vi "CriticalMain.vi"(8 "error in (no error)":errorcluster) -> (0 "error out":errorcluster)   [LabVIEW 2014]
uses:
  Type Defs/CriticalToFValues.ctl
  Type Defs/PositionSensorData.ctl
  Type Defs/PodState.ctl
  <vilib>/Platform/TimedLoop/XDataNode/timing_clust.ctl
  <vilib>/Platform/TimedLoop/XDataNode/nitl_modes.ctl
  <vilib>/Platform/TimedLoop/XDataNode/wakeup.ctl
  <vilib>/myRIO/Instrument Drivers/Onboard Devices/Accelerometer/typedefs/Accelerometer Reference.ctl
  <vilib>/myRIO/Common/Instrument Driver Framework/Utilities/typedefs/myRIO Generic Hardware Reference.ctl
  <vilib>/myRIO/Common/Instrument Driver Framework/Utilities/typedefs/Hardware Version Enum.ctl
  <vilib>/myRIO/Common/Instrument Driver Framework/Utilities/typedefs/myRIO v1.0 Reference.ctl
  <vilib>/myRIO/Common/Instrument Driver Framework/Utilities/typedefs/Generic FPGA Reference.ctl
  <vilib>/myRIO/Common/Instrument Driver Framework/myRIO v1.0/Accelerometer/typedefs/Accelerometer Channels List.ctl
  <vilib>/myRIO/Common/Instrument Driver Framework/myRIO v1.0/Accelerometer/typedefs/Accelerometer Channels Enum.ctl
  <vilib>/userdefined/High Color/nirio_resource_hc.ctl
  <vilib>/myRIO/Instrument Drivers/Onboard IO/DIO/typedefs/DIO Reference.ctl
  <vilib>/myRIO/Common/Instrument Driver Framework/myRIO v1.0/DIO/typedefs/DIO Channels List.ctl
  <vilib>/myRIO/Common/Instrument Driver Framework/myRIO v1.0/DIO/typedefs/DIO Channels Enum.ctl
  <vilib>/myRIO/Common/Instrument Driver Framework/Utilities/vis/Is FPGA Ref Available.vi
  <vilib>/myRIO/Common/Instrument Driver Framework/myRIO v1.0/Accelerometer/vis/myRIO v1.1 Open Accelerometer.vi
  <vilib>/myRIO/Instrument Drivers/Onboard Devices/Accelerometer/vis/Read.vi
  <vilib>/myRIO/Common/Instrument Driver Framework/myRIO v1.0/DIO/vis/myRIO v1.1 Open DIO.vi
  <vilib>/myRIO/Instrument Drivers/Onboard IO/DIO/vis/Read.vi
  <vilib>/MakerHub/LINX/Public/Peripherals/Digital/Digital Write N Chans.vi
  <vilib>/myRIO/Common/Instrument Driver Framework/Utilities/vis/Validate Channels.vi
  <vilib>/myRIO/Common/Instrument Driver Framework/myRIO v1.0/Accelerometer/vis/myRIO v1.0 Reserve Accelerometer.vi
  <vilib>/myRIO/Common/Instrument Driver Framework/myRIO v1.0/DIO/vis/myRIO v1.0 Reserve DIO.vi
  <vilib>/MakerHub/LINX/Private/Local IO/LinxDigitalWrite.vi
  <vilib>/MakerHub/LINX/Public/Utilities/Check Channel.vi
  <vilib>/myRIO/Common/Instrument Driver Framework/myRIO v1.0/Resource Manager/vis/myRIO v1.0 Reserve Channel List.vi
  <vilib>/myRIO/Common/Instrument Driver Framework/myRIO v1.0/Accelerometer/vis/myRIO v1.0 Build MUX Configuration Accelerometer.vi
  <vilib>/myRIO/Common/Instrument Driver Framework/myRIO v1.0/DIO/vis/myRIO v1.0 Build MUX Configuration DIO.vi
  <vilib>/MakerHub/LINX/Private/myRIO/Utilities/Get DIO Channel Name.vi
  <vilib>/myRIO/Common/Instrument Driver Framework/myRIO v1.0/Resource Manager/vis/myRIO v1.0 Reserve Channel.vi
  <vilib>/myRIO/Common/Instrument Driver Framework/myRIO v1.0/Resource Manager/vis/myRIO v1.0 Unreserve Channel.vi
  <vilib>/myRIO/Common/Instrument Driver Framework/myRIO v1.0/Resource Manager/vis/myRIO v1.0 Create Configuration List.vi
  <vilib>/myRIO/Common/Instrument Driver Framework/myRIO v1.0/Resource Manager/vis/myRIO v1.0 Build Mutex Name.vi
  <vilib>/MakerHub/LINX/Public/Utilities/Open Local.vi
  <vilib>/Platform/TimedLoop/scheduler/LVUserAPI/_suppVIs/Create_1kHz_TSource.vi
  <vilib>/MakerHub/LINX/Private/Utilties/Generate Error.vi
  <vilib>/Utility/VariantDataType/GetNumericInfo.vi
  <vilib>/Utility/error.llb/Error Cluster From Error Code.vi
  <vilib>/myRIO/Common/Instrument Driver Framework/myRIO v1.0/myRIO v1.1 Open.vi
  <vilib>/myRIO/Common/Instrument Driver Framework/myRIO v1.0/Accelerometer/vis/myRIO v1.0 Get Scaling Constant Accelerometer.vi
  <vilib>/myRIO/Common/Instrument Driver Framework/Utilities/vis/IO Manager.vi
  <vilib>/myRIO/Common/Instrument Driver Framework/Utilities/vis/Configuration Manager.vi
  <vilib>/myRIO/Common/Instrument Driver Framework/myRIO v1.0/myRIO v1.0 Close.vi
  <vilib>/myRIO/Common/Instrument Driver Framework/myRIO v1.0/Accelerometer/vis/myRIO v1.0 Read Accelerometer.vi
  <vilib>/myRIO/Common/Instrument Driver Framework/myRIO v1.0/Resource Manager/vis/myRIO v1.0 Configure IO.vi
  <vilib>/myRIO/Common/Instrument Driver Framework/myRIO v1.0/DIO/vis/myRIO v1.0 Read DIO.vi
  <vilib>/platform/TimedLoop/XDataNode/XDataNode.xnode
  <vilib>/myRIO/Express VI/Onboard Devices/Accelerometer/Accelerometer Express VI.xnode
  <vilib>/myRIO/Instrument Drivers/Onboard Devices/Accelerometer/vis/myRIO Accelerometer Open.xnode
  <vilib>/myRIO/Express VI/Onboard IO/DI/DI Express VI.xnode
  <vilib>/myRIO/Instrument Drivers/Onboard IO/DIO/vis/myRIO DIO Open.xnode
  <vilib>/Platform/TimedLoop/XDataNode/XDNodeRunTimeDep.lvlib
  <vilib>/myRIO/Instrument Drivers/Onboard IO/DIO/DIO.lvlib
  <vilib>/MakerHub/LINX/LMH-LINX.lvlib
  <vilib>/myRIO/Instrument Drivers/Onboard Devices/Accelerometer/Accelerometer.lvlib
panel:
  in  "Release Friction Brakes":bool
  in  "Release Magnetic Brakes":bool
  in  "Force Brakes Close":bool
  in  "Open Brakes":bool
  in  "Levitate":bool
  out "Position Data Lost":u32
  out "ToF Data Lost":u32
  out "Position Sensor Data":T1
  out "Accelerometer Error":bool
  out "Critical ToF Values":T2
  in  "Speed Read":bool
  out "Attempts":i32
  out "Sensor Error Code":u8
  in  "Attempts before Timeout":u16=10
  out "Laser Error":bool
  in  "Reset":bool
  in  "Stop":bool
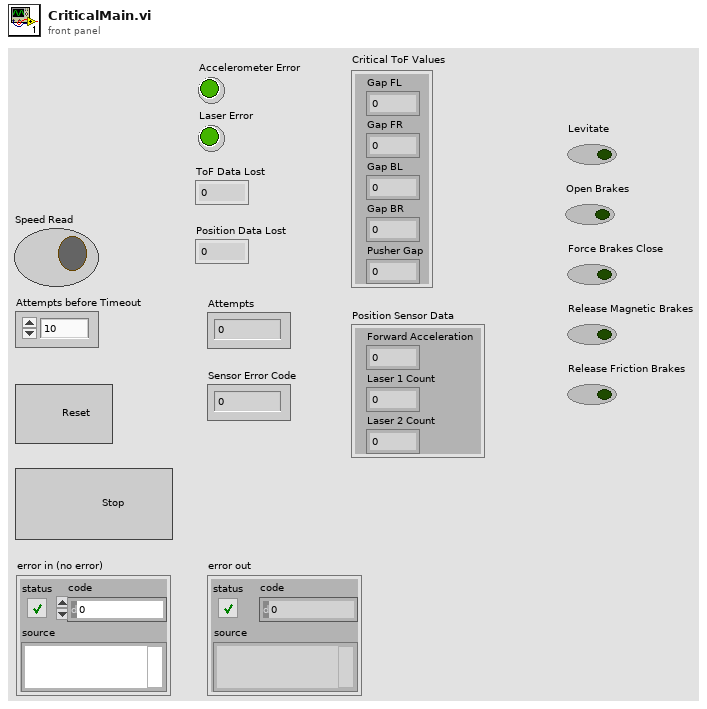
[diagram p1: front panel]
types:
  T1 = typedef "PositionSensorData.ctl" = cluster{"Forward Acceleration":i16, "Laser 1 Count":u16, "Laser 2 Count":u16}
  T2 = typedef "CriticalToFValues.ctl" = cluster{"Gap FL":u8, "Gap FR":u8, "Gap BL":u8, "Gap BR":u8, "Pusher Gap":u8}
  T3 = cluster{"read mode":enum16{"polling", "blocking"}, "write mode":enum16{"polling", "blocking"}}
  T4 = typedef "PodState.ctl" = enum8{"PreFlight", "Accelerating", "Coast", "Brake", "PostFlight"}
  T5 = typedef "LMH-LINX.lvlib/LINX Ref.ctl" = cluster{"IO":T6, "Interface":T7, "LINX Device Config":T8}
  T6 = typedef "LMH-LINX.lvlib/Platform.ctl" = enum16{"Remote", "Local"}
  T7 = typedef "LMH-LINX.lvlib/Interface.ctl" = enum16{"Serial", "TCP"}
  T8 = typedef "LMH-LINX.lvlib/Device.lvlib/LINX Device Config.ctl" = cluster{"Interface":T7, "COM Port":refnum<visa-resource-name>, "TCP Configuration":T9, "Device Family":u8, "Device ID":u8, "Device Name":string, "TCP Ref":refnum<k5>, "Channels":T10}
  T9 = typedef "LMH-LINX.lvlib/Device.lvlib/TCP Config.ctl" = cluster{"IP Address":string, "Port":u16}
  T10 = typedef "LMH-LINX.lvlib/Channels.ctl" = cluster{"DI":u8[], "DO":u8[], "AI":u8[], "AO":u8[], "PWM":u8[], "QE":u8[], "UART":u8[], "I2C 2":u8[], "SPI":u8[], "CAN":u8[], "Servo":u8[], "AI Ref (V)":dbl, "AI Resolution (Bits)":u8, "AO Ref (V)":dbl, "AO Resolution (Bits)":u8}
  T11 = typedef "VL6180 Resource.ctl" = cluster{"I2C Channel":u8, "I2C Slave Address":u8, "Online":bool}
  T12 = typedef "XDNodeRunTimeDep.lvlib/timing_clust.ctl" = cluster{"Expected End [f-1]":u64, "Actual End [f-1]":u64, "Finished Late? [f-1]":bool, "Expected End [i-1]":u64, "Actual End [i-1]":u64, "Finished Late? [i-1]":bool, "Expected Start [i]":u64, "Actual Start [i]":u64, "Expected Start [f]":u64, "Actual Start [f]":u64, "Source Name":string, "Structure Name":string, "Period":i64, "Deadline":i64, "Offset":i64, "Start":i64, "Priority":i32, "Timeout":i32, "Mode":T13, "Wakeup Reason":T14, "Error":errorcluster, "Source Type":string, "Secondary Source Type":string, "Global End Time":u64, "Global Start Time":u64, "Frame Duration":u64, "Iteration Duration":u64, "Assigned CPU":i32, "I/O Scan Engine Mode":u32}
  T13 = typedef "XDNodeRunTimeDep.lvlib/nitl_modes.ctl" = enum32{"No Change", "Process missed periods, maintain original phase", "Discard missed periods, maintain original phase", "Process missed periods, ignore original phase", "Discard missed periods, ignore original phase"}
  T14 = typedef "XDNodeRunTimeDep.lvlib/wakeup.ctl" = enum32{"Normal", "Aborted", "Asynchronous wakeup", "Timing source error", "Timed loop error", "Timeout"}
  T15 = typedef "Accelerometer.lvlib/Accelerometer Reference.ctl" = cluster{"myRIO Reference":T16, "Accelerometer Channels List":T20, "LSB Weight":dbl}
  T16 = typedef "myRIO Generic Hardware Reference.ctl" = cluster{"myRIO Model":T17, "myRIO Hardware Reference":T18}
  T17 = typedef "Hardware Version Enum.ctl" = enum16{"Unknown", "myRIO-1900", "myRIO-1950"}
  T18 = typedef "myRIO v1.0 Reference.ctl" = cluster{"Generic FPGA Reference":T19, "Allow multiple opens":bool}
  T19 = typedef "Generic FPGA Reference.ctl" = refnum<k20>
  T20 = typedef "Accelerometer Channels List.ctl" = T21[]
  T21 = typedef "Accelerometer Channels Enum.ctl" = enum16{"Not Connected", "X-Axis", "Y-Axis", "Z-Axis"}
  T22 = typedef "nirio_resource_hc.ctl" = tag
  T23 = typedef "DIO.lvlib/DIO Reference.ctl" = cluster{"myRIO Reference":T16, "DIO Channels List":T24}
  T24 = typedef "DIO Channels List.ctl" = T25[]
  T25 = typedef "DIO Channels Enum.ctl" = enum16{"Not Connected", "C/DIO0", "C/DIO1", "C/DIO2", "C/DIO3", "C/DIO4", "C/DIO5", "C/DIO6", "C/DIO7", "A/DIO0", "A/DIO1", "A/DIO2", "A/DIO3", "A/DIO4", "A/DIO5", "A/DIO6", "A/DIO7", "A/DIO8", "A/DIO9", "A/DIO10", "A/DIO11", "A/DIO12", "A/DIO13", "A/DIO14", "A/DIO15", "B/DIO0", "B/DIO1", "B/DIO2", "B/DIO3", "B/DIO4", "B/DIO5", "B/DIO6", "B/DIO7", "B/DIO8", "B/DIO9", "B/DIO10", "B/DIO11", "B/DIO12", "B/DIO13", "B/DIO14", "B/DIO15", "LED0", "LED1", "LED2", "LED3", "Button0"}
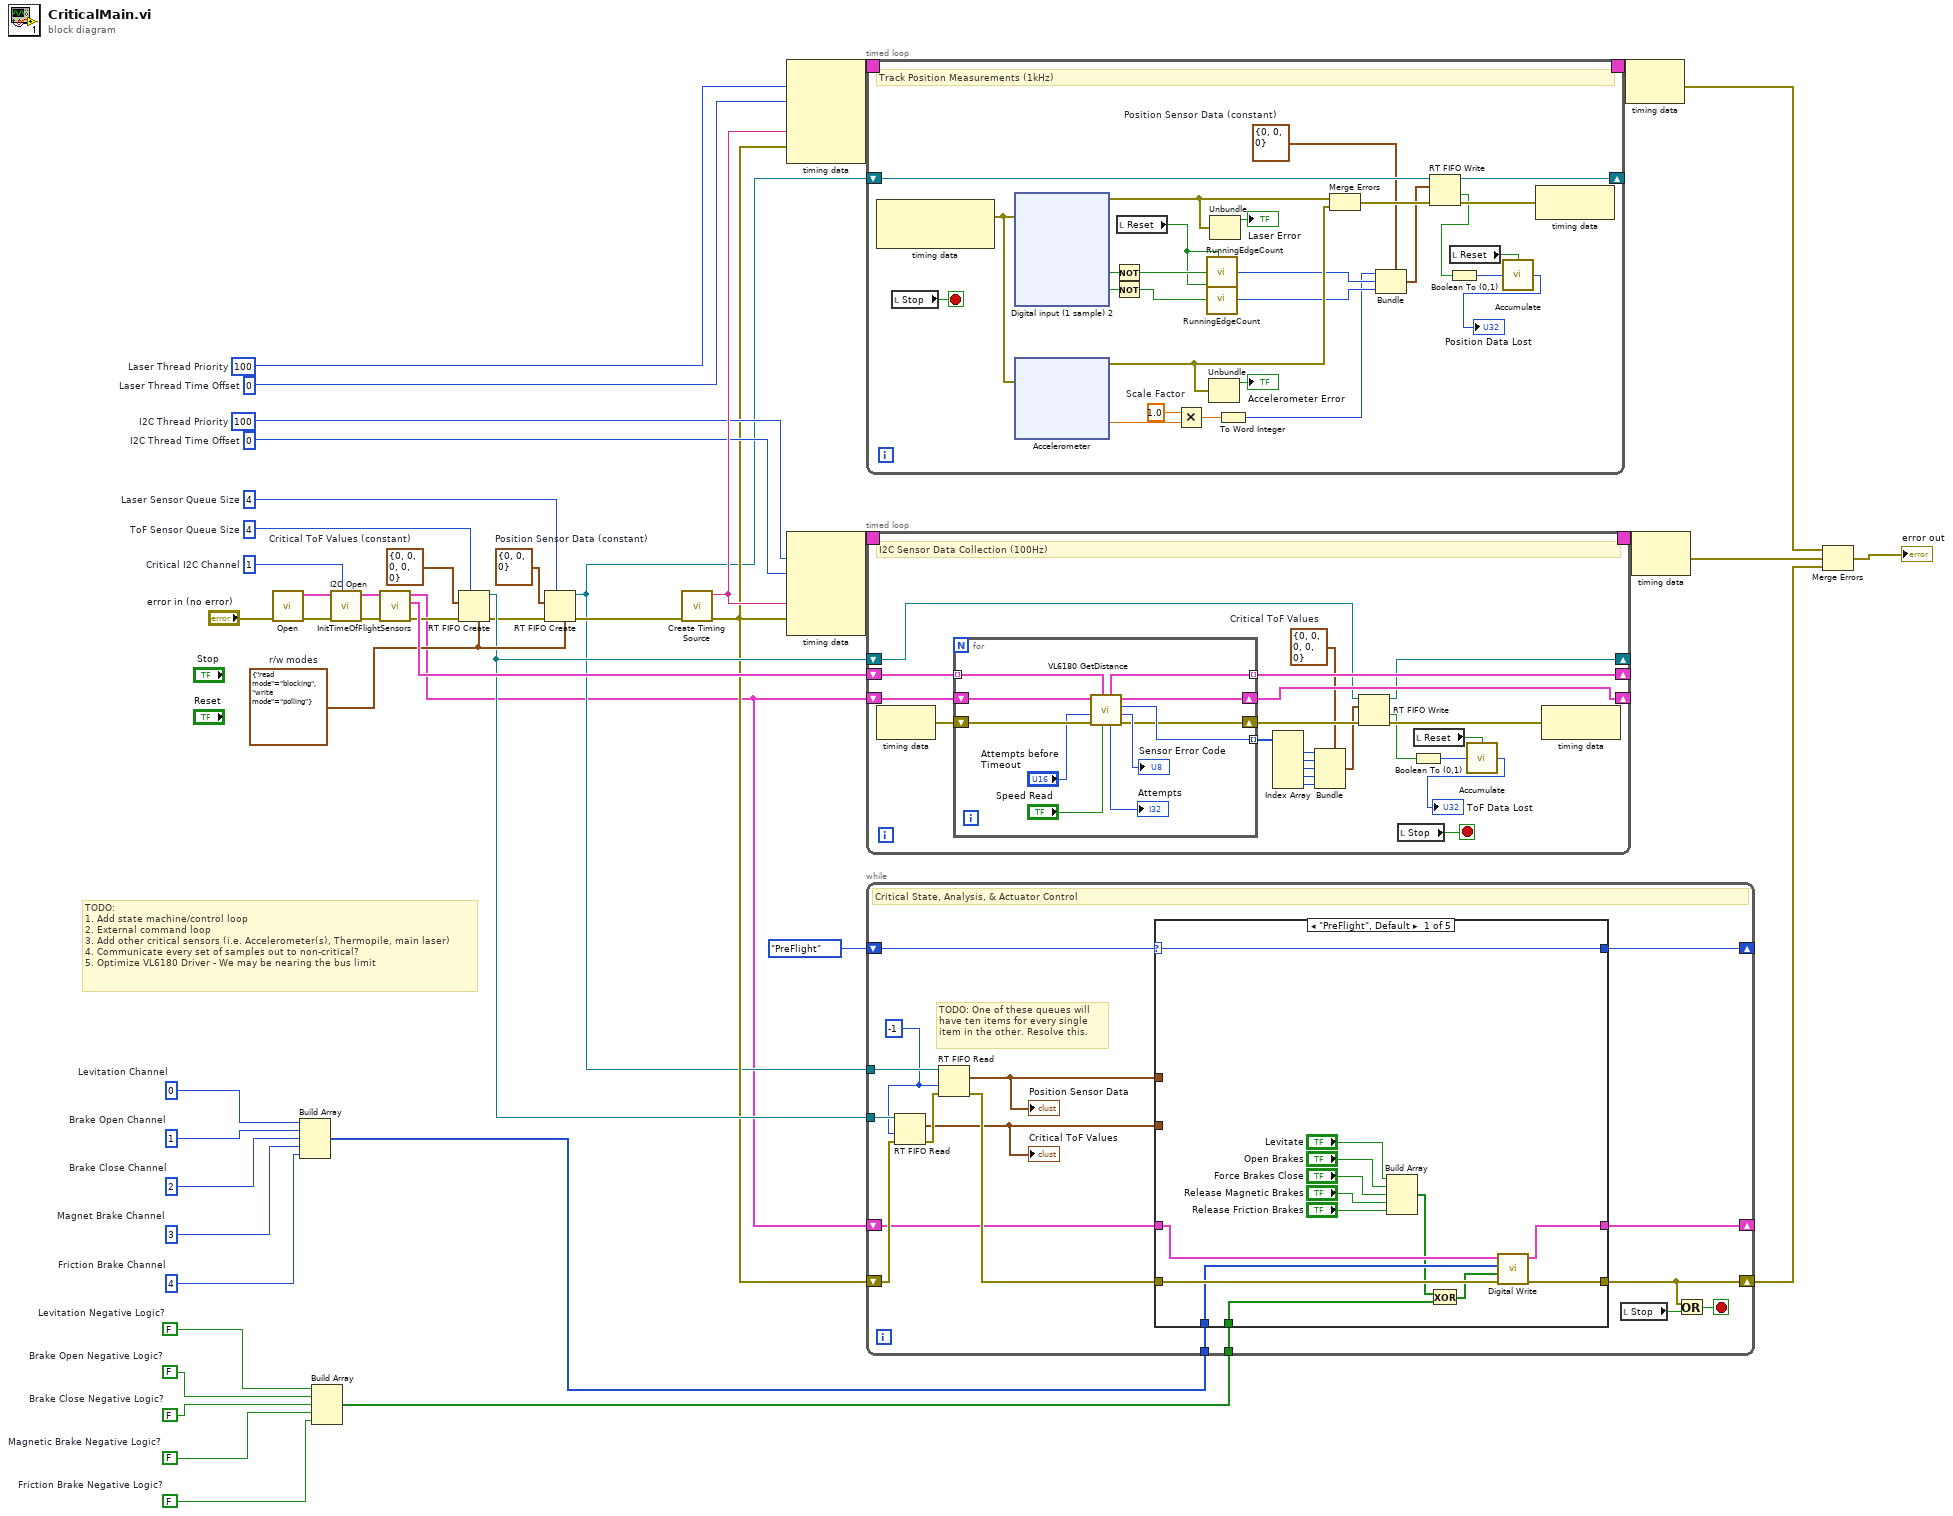
[diagram p0: block diagram]
diagram:
  w5 = FALSE  # Brake Open Negative Logic?
  w4 = FALSE  # Brake Close Negative Logic?
  w2 = FALSE  # Magnetic Brake Negative Logic?
  w3 = FALSE  # Friction Brake Negative Logic?
  w6 = FALSE  # Levitation Negative Logic?
  w11 = u8 1  # Brake Open Channel
  w10 = u8 2  # Brake Close Channel
  w9 = u8 3  # Magnet Brake Channel
  w8 = u8 4  # Friction Brake Channel
  w12 = u8 0  # Levitation Channel
  w24 = T3 {"read mode"=enum."blocking", "write mode"=enum."polling"}  # r/w modes
  w14 = T1 {"Forward Acceleration"=0, "Laser 1 Count"=0, "Laser 2 Count"=0}  # Position Sensor Data (constant)
  w16 = 4  # Laser Sensor Queue Size
  w26 = T2 {"Gap FL"=0, "Gap FR"=0, "Gap BL"=0, "Gap BR"=0, "Pusher Gap"=0}  # Critical ToF Values (constant)
  w25 = 4  # ToF Sensor Queue Size
  w28 = i64 0  # I2C Thread Time Offset
  w29 = 100  # I2C Thread Priority
  w30 = i64 0  # Laser Thread Time Offset
  w31 = 100  # Laser Thread Priority
  w40 = u8 1  # Critical I2C Channel
  # "TODO:\n1. Add state machine/control loop\n2. External command loop\n3. Add other critical sensors (i.e. Accelerometer(s), Thermopile, main laser)\n4. Communicate every set of samples out to non-critical?\n5. Optimize VL6180 Driver - We may be nearing the bus limit"
  n1 = call-poly <vilib>:"Open.vi"("Error In"="error in (no error)") -> ("Error Out"=w41:errorcluster, "LINX Resource"=w42:T5)  [unwired: 8 in, 1 out]
  n2 = Build Array(w12, w11, w10, w9, w8) -> (w7:u8[])
  n3 = Build Array(w6, w5, w4, w2, w3) -> (w1:bool[])
  n4 = call <vilib>:"I2C Open.vi"("I2C Channel (0)"=w40, "Error In"=w41, "LINX Resource"=w42) -> ("Error Out"=w39:errorcluster, "LINX Resource"=w38:T5)  [unwired: 7 in]
  n5 = call "InitTimeOfFlightSensors.vi"("error in (no error)"=w39, "LINX Resource"=w38) -> ("error out"=w27:errorcluster, "VL6180 Resources"=w34:T11[], "LINX Resource Out"=w13:T5)  [unwired: 7 in]
  n6 = RT FIFO Create(1:w26, 3:w27, 4:w25, 7:w24) -> (8:w23:refnum<k33>, 11:w18:errorcluster)  [unwired: 4 in, 1 out]
  n7 = RT FIFO Create(1:w14, 3:w18, 4:w16, 7:w24) -> (8:w15:refnum<k33>, 11:w17:errorcluster)  [unwired: 4 in, 1 out]
  n8 = call-poly <vilib>:"Create Timing Source.vi"("error in (no error)"=w17) -> ("error out"=w21:errorcluster, "name (out)"=w35:string)  [unwired: 9 in]
  n9 = node-c288(w31, w30, w35, w21) -> (w45:T12)  [unwired: 1 in]
  n10 = node-c288(w29, w28, w35, w21) -> (w37:T12)  [unwired: 1 in]
  n11 = timed-loop {
    timing: w45 -> [_]
    timing-out: [_] -> w44
    shift-right: [w46] -> _
    shift-left: w15 -> [w64]
    stop <- w67 stop-if-true
    w57 = T1 {"Forward Acceleration"=0, "Laser 1 Count"=0, "Laser 2 Count"=0}  # Position Sensor Data (constant)
    w62 = 1.0  # Scale Factor
    # "Track Position Measurements (1kHz)"
    n12 = node-c288() -> (w58:errorcluster)  [unwired: 1 in, 1 out]
    n13 = local read "Stop"() -> (w67:bool)
    n14 = xnode "Digital input (1 sample) 2"("error in (no error)"=w58) -> ("Laser 1 (A/DIO0 (Pin 11))"=w70:bool, "Laser 2 (A/DIO1 (Pin 13))"=w69:bool, "error out"=w52:errorcluster)
    n15 = xnode "Accelerometer"("error in (no error)"=w58) -> ("Back"=w63:dbl, "error out"=w71:errorcluster)  [unwired: 2 out]
    n16 = Not(x=w70) -> (.not. x?=w60:bool)
    n17 = Not(x=w69) -> (.not. x?=w68:bool)
    n18 = local read "Reset"() -> (w51:bool)
    n19 = Multiply(x=w62, y=w63) -> (x*y=w61:dbl)
    n20 = call "RunningEdgeCount.vi"("Reset Count? (F)"=w51, "Input"=w60) -> ("Count"=w56:u32)  [unwired: 3 in]
    n21 = call "RunningEdgeCount.vi"("Reset Count? (F)"=w51, "Input"=w68) -> ("Count"=w55:u32)  [unwired: 3 in]
    n22 = Unbundle(w71) -> ("status"=→"Accelerometer Error":bool)  [unwired: 2 out]
    n23 = Unbundle(w52) -> ("status"=→"Laser Error":bool)  [unwired: 2 out]
    n24 = To Word Integer(number=w61) -> (16bit integer=w54:i16)
    n25 = Merge Errors(w52, w71) -> (w72:errorcluster)
    n26 = Bundle(cluster=w57, "Forward Acceleration"=w54, "Laser 1 Count"=w56, "Laser 2 Count"=w55) -> (w53:T1)
    n27 = RT FIFO Write(0:w64, 1:w53, 3:w72) -> (8:w46:refnum<k33>, 10:w50:bool, 11:w65:errorcluster)  [unwired: 2 in, 1 out]
    n28 = Boolean To (0,1)(Boolean=w50) -> (0, 1=w49:i16)
    n29 = local read "Reset"() -> (w48:bool)
    n30 = call "Accumulate.vi"("Input"=w49, "Reset? (F)"=w48) -> ("Accumulation"=→"Position Data Lost":i32)
    n31 = node-c288(w65) -> ()  [unwired: 1 out]
  }
  n32 = timed-loop {
    timing: w37 -> [_]
    timing-out: [_] -> w36
    shift-right: [w170] -> _
    shift-left: w34 -> [w173]
    shift-right: [w161] -> _
    shift-left: w13 -> [w172]
    shift-right: [w160] -> _
    shift-left: w23 -> [w159]
    stop <- w169 stop-if-true
    w158 = T2 {"Gap FL"=0, "Gap FR"=0, "Gap BL"=0, "Gap BR"=0, "Pusher Gap"=0}  # Critical ToF Values
    # "I2C Sensor Data Collection (100Hz)"
    n33 = node-c288() -> (w171:errorcluster)  [unwired: 1 in]
    n34 = for {
      tunnel: [w181] -> w170 mode=indexing
      shift-right: [w179] -> w161
      shift-left: w172 -> [w180]
      tunnel: w173 -> [w175] mode=indexing
      tunnel: [w178] -> w174 mode=indexing
      shift-right: [w177] -> w163
      shift-left: w171 -> [w185]
      n35 = call "VL6180 GetDistance.vi"("Speed Read"="Speed Read", "VL6180 Resource in"=w175, "error in (no error)"=w185, "Attempts before Timeout"="Attempts before Timeout", "LINX Resource"=w180) -> ("error out"=w177:errorcluster, "Sensor Error Code"=→"Sensor Error Code":u8, "Distance (mm)"=w178:u8, "LINX Resource"=w179:T5, "Attempts"=→"Attempts":i32, "VL6180 Resource out"=w181:T11)  [unwired: 1 in]
    }
    n36 = Index Array(array=w174) -> (element #1=w168:u8, element #2=w167:u8, element #3=w166:u8, element #4=w165:u8, element #5=w164:u8)  [unwired: 5 in]
    n37 = Bundle(cluster=w158, "Gap FL"=w168, "Gap FR"=w167, "Gap BL"=w166, "Gap BR"=w165, "Pusher Gap"=w164) -> (w162:T2)
    n38 = RT FIFO Write(0:w159, 1:w162, 3:w163) -> (8:w160:refnum<k33>, 10:w154:bool, 11:w157:errorcluster)  [unwired: 2 in, 1 out]
    n39 = local read "Stop"() -> (w169:bool)
    n40 = Boolean To (0,1)(Boolean=w154) -> (0, 1=w155:i16)
    n41 = local read "Reset"() -> (w156:bool)
    n42 = call "Accumulate.vi"("Input"=w155, "Reset? (F)"=w156) -> ("Accumulation"=→"ToF Data Lost":i32)
    n43 = node-c288(w157) -> ()  [unwired: 1 out]
  }
  n44 = while {
    tunnel: w23 -> [w206]
    shift-right: [w204] -> _
    shift-left: PodState."PreFlight" ("PodState") -> [w207]
    shift-right: [w201] -> w19
    shift-left: w21 -> [w205]
    tunnel: w15 -> [w197]
    tunnel: w7 -> [w193]
    tunnel: w1 -> [w192]
    shift-right: [w191] -> _
    shift-left: w13 -> [w194]
    stop <- w202 stop-if-true
    w195 = -1 ("timeout in ms (0)")
    # "TODO: One of these queues will\nhave ten items for every single\nitem in the other. Resolve this."
    # "Critical State, Analysis, & Actuator Control"
    n45 = RT FIFO Read(0:w206, 2:w195, 3:w205) -> (9:w198:T2, 11:w200:errorcluster)  [unwired: 1 in, 3 out]
    "Critical ToF Values" <- w198
    n46 = RT FIFO Read(0:w197, 2:w195, 3:w200) -> (9:w196:T1, 11:w199:errorcluster)  [unwired: 1 in, 3 out]
    "Position Sensor Data" <- w196
    n47 = case shown="\"PreFlight\", Default" w207 {
      selector: w207 -> [w221 w223 w226 w229 w232]
      tunnel: [w221 w223 w226 w229 w232] -> w204
      tunnel: [w217 w224 w227 w230 w233] -> w201
      tunnel: w199 -> [w220 w224 w227 w230 w233]
      tunnel: w198 -> [_ _ _ _ _]
      tunnel: w196 -> [_ _ _ _ _]
      tunnel: w194 -> [w219 w222 w225 w228 w231]
      tunnel: w193 -> [w218 _ _ _ _]
      tunnel: w192 -> [w208 _ _ _ _]
      tunnel: [w215 w222 w225 w228 w231] -> w191
      frame "PreFlight", Default {
        n48 = Build Array("Levitate", "Open Brakes", "Force Brakes Close", "Release Magnetic Brakes", "Release Friction Brakes") -> (w209:bool[])
        n49 = Exclusive Or(1:w208, 2:w209) -> (0:w216:bool[])
        n50 = call-poly <vilib>:"Digital Write.vi"("Error In"=w220, "Values"=w216, "DO Channels"=w218, "LINX Resource"=w219) -> ("Error Out"=w217:errorcluster, "LINX Resource"=w215:T5)  [unwired: 6 in]
      }
      frame "Accelerating" {
      }
      frame "Coast" {
      }
      frame "Brake" {
      }
      frame "PostFlight" {
      }
    }
    n51 = local read "Stop"() -> (w203:bool)
    n52 = Or(x=w201, y=w203) -> (x .or. y?=w202:bool)
  }
  n53 = node-c288(w44) -> (w32:errorcluster)
  n54 = node-c288(w36) -> (w33:errorcluster)
  n55 = Merge Errors(w32, w33, w19) -> (→"error out":errorcluster)
